vi "Database.WriteStationValues.vi"(8 "error in":errorcluster, 10 "FileName":string, 11 "Data in":T1 {"Variant"."TS"."TV"."minimum" format="%#.3f"; "Variant"."TS"."TV"."maximum" format="%#.3f"; "Variant"."TS"."TP"."value" format="%#.3f"}) -> (0 "error out":errorcluster, 3 "Data out":T1 {"Variant"."TS"."TV"."minimum" format="%#.3f"; "Variant"."TS"."TV"."maximum" format="%#.3f"; "Variant"."TS"."TP"."value" format="%#.3f"})   [LabVIEW 2016]
doc: "Write test results (measurement values) to proda database\n\nWabco 2017 All right reserved\nAuthor: maciej.szupienko@wabco-auto.com"
uses:
  tools/Translator/Translator.Message.ctl
  tools/EventLog/EventLog.EventSource.ctl
  Global/ApplicationGlobal.vi
  tools/EventLog/EventLog.New(single).vi
  Database.Main.Data.Sets.ctl
  Database.Main.Data.Status.ctl
  ProdaNG/Controls/ProdaNG.ProcessResult.ctl
  ProdaNG/Controls/ProdaNG.ProcessStepResult.ctl
  ProdaNG/Controls/ProdaNG.TestStepResult.ctl
  ProdaNG/Controls/ProdaNG.TestValueResult.ctl
  ProdaNG/Controls/ProdaNG.Identification.ctl
  Database.Main.Data.ctl
  Database.Main.Data.Results.ctl
  ProdaNG/Controls/ProdaNG.TestStepParam.ctl
  ProdaNG/Controls/ProdaNG.TestValue.ctl
  ProdaNG/Controls/ProdaNG.TestStep.ctl
  ProdaNG/Controls/ProdaNG.ProcessStepParam.ctl
  Database.Main.Data.Variant.ctl
panel:
  out "Prod saved":bool
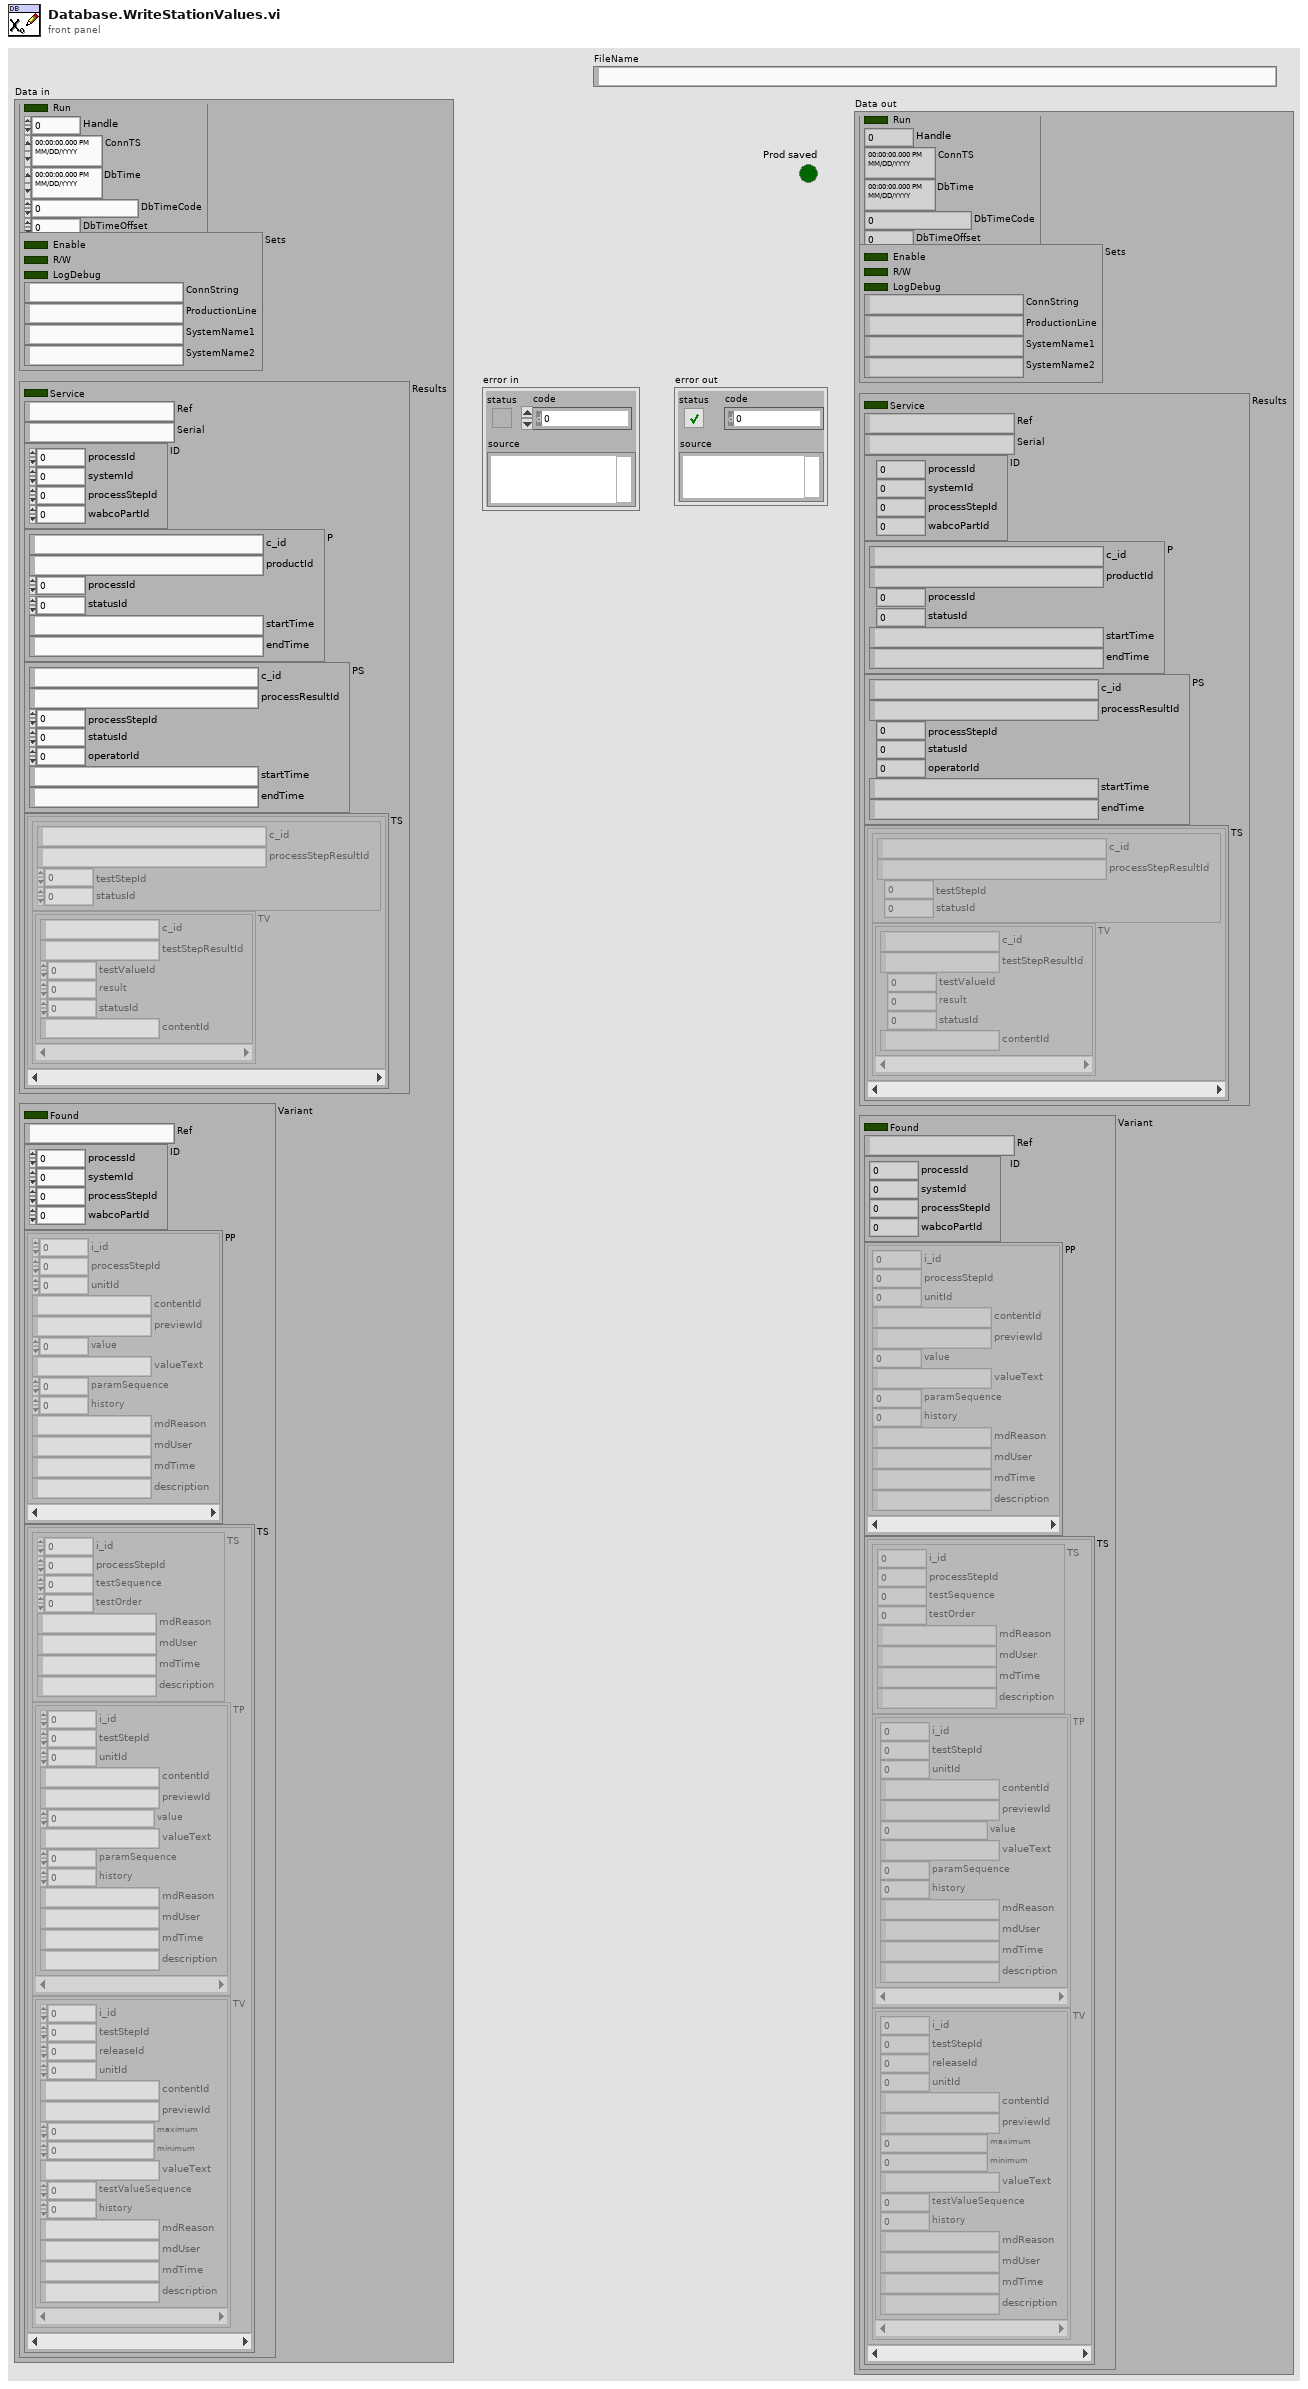
[diagram p1: front panel]
types:
  T1 = typedef "Database.Main.Data.ctl" = cluster{"Status":T2, "Sets":T3, "Results":T4, "Variant":T10}
  T2 = typedef "Database.Main.Data.Status.ctl" = cluster{"Run":bool, "Handle":i32, "ConnTS":timestamp, "DbTime":timestamp, "DbTimeCode":dbl, "DbTimeOffset":dbl}
  T3 = typedef "Database.Main.Data.Sets.ctl" = cluster{"Enable":bool, "R/W":bool, "LogDebug":bool, "ConnString":string, "ProductionLine":string, "SystemName1":string, "SystemName2":string}
  T4 = typedef "Database.Main.Data.Results.ctl" = cluster{"Service":bool, "Ref":string, "Serial":string, "ID":T5, "P":T6, "PS":T7, "TS":cluster{"TS":T8, "TV":T9[]}[]}
  T5 = typedef "ProdaNG.Identification.ctl" = cluster{"processId":i32, "systemId":i32, "processStepId":i32, "wabcoPartId":i32}
  T6 = typedef "ProdaNG.ProcessResult.ctl" = cluster{"c_id":string, "productId":string, "processId":i32, "statusId":i32, "startTime":string, "endTime":string}
  T7 = typedef "ProdaNG.ProcessStepResult.ctl" = cluster{"c_id":string, "processResultId":string, "processStepId":i32, "statusId":i32, "operatorId":i32, "startTime":string, "endTime":string}
  T8 = typedef "ProdaNG.TestStepResult.ctl" = cluster{"c_id":string, "processStepResultId":string, "testStepId":i32, "statusId":i32}
  T9 = typedef "ProdaNG.TestValueResult.ctl" = cluster{"c_id":string, "testStepResultId":string, "testValueId":i32, "result":dbl, "statusId":i32, "contentId":string}
  T10 = typedef "Database.Main.Data.Variant.ctl" = cluster{"Found":bool, "Ref":string, "ID":T5, "PP":T11[], "TS":cluster{"TS":T12, "TP":T13[], "TV":T14[]}[]}
  T11 = typedef "ProdaNG.ProcessStepParam.ctl" = cluster{"i_id":i32, "processStepId":i32, "unitId":i32, "contentId":string, "previewId":string, "value":dbl, "valueText":string, "paramSequence":i32, "history":i32, "mdReason":string, "mdUser":string, "mdTime":string, "description":string}
  T12 = typedef "ProdaNG.TestStep.ctl" = cluster{"i_id":i32, "processStepId":i32, "testSequence":i32, "testOrder":i32, "mdReason":string, "mdUser":string, "mdTime":string, "description":string}
  T13 = typedef "ProdaNG.TestStepParam.ctl" = cluster{"i_id":i32, "testStepId":i32, "unitId":i32, "contentId":string, "previewId":string, "value":dbl, "valueText":string, "paramSequence":i32, "history":i32, "mdReason":string, "mdUser":string, "mdTime":string, "description":string}
  T14 = typedef "ProdaNG.TestValue.ctl" = cluster{"i_id":i32, "testStepId":i32, "releaseId":i32, "unitId":i32, "contentId":string, "previewId":string, "maximum":dbl, "minimum":dbl, "valueText":string, "testValueSequence":i32, "history":i32, "mdReason":string, "mdUser":string, "mdTime":string, "description":string}
  T15 = typedef "EventLog.EventSource.ctl" = enum16{"All", "Gui", "Ref", "File", "Arch", "Seq", "CPX", "DB", "Laser", "Scan.P", "Scan.O"}
  T16 = typedef "Translator.Message.ctl" = enum16{"-", "Event confirmed", "Log out", "Log in", "Shutdown", "Cancel", "Start", "Begin time", "End time", "Duration", "Service Mode", "Ignore Results", "Serial Format", "On", "Off", "OK", "NOK", "NOK %s", "Home", "Work", "Close", "Open", "In progress...", "Missing", "Empty", "Hardware failure", "Initial", "Default", "Total", "Out of range", "Free disk space is below 1GB - contact technician", "Error %d >> %s", "Error %d >> %s >> %s", "Msg %d >> %s", "Laser msg %d %s", "Laser cmd error %s %d", "Laser cmd failed %s", "Laser cmd warning %s", "Laser disconnected", "Laser status %s", "Laser already started", "Laser job unkonwn %s", "Laser job missing %s", "Laser job select failure %s", "Unable to start laser printing (%s)", "Unable to stop laser printing (%s)", "Laser marking aborted", "Laser marking timeout", "Unable to reset Laser Interlock (%s)", "Unable to trigger Laser. Laser not ready (%s)", "Laser job '%s' coordinates not configured", "Starting %s", "Quitting %s", "Configured", "Initializing", "Quitting", "Loading", "Loaded %d results", "Loaded %d events", "Running", "Stopped", "Summary", "Laser", "Do you want to continue?", "Do you want to delete the configuration?", "The configuration is being used by an order. Unable to delete!", "Press confirm button", "Station is not based. Do you want to exit?", "Station requires changeover. Do you want to run the test?", "Test options are not set as default. Do you want to continue?", "Formatting of WabcoNo is disabled. Do you want to continue?", "Product not detected. Do you want to continue?", "Product scan failed. Do you want to continue?", "Calibration", "Log out?", "System", "All", "IDLE", "Translating...%s", "Not found", "Alarm %s", "Run", "Skip", "Abort", "Repeat", "Please wait...", "Database disconnected", "Database disconnected - changeover disabled!", "Login to database successful", "Login to database failed: %d; %s", "Unable to check the product status of reference %d - database disconnected", "Unable to set the product status of reference %d - database disconnected", "Variant file backup %s", "Read variant (%s)", "Result", "Station armed!", "Station requires changeover!", "Select reference number...", "EMERGENCY BUTTON - press Control button", "EMERGENCY DOOR - press Control button", "Resetting Emergency...", "Unable to reset safety circuit - Emergency Button pressed", "Unable to reset safety circuit - Emergency Side Door open", "Station not based", "Station based", "Station not empty", "Station basing...", "No order", "Press Start to begin new order", "Scanning new order", "Order NOK. Correct or scan again", "Order OK. Press Accept", "Order ready", "Revolver incorrect", "Fork incorrect", "Revolver missing", "Revolver empty", "Container missing", "Offline results", "Offline statistics", "Updating statistics %.1f %%", "DMC Configurator", "Door open", "Close the front door", "Press start button", "Done. Open the front door", "Running...", "Running...%.1f %%", "Pause %s", "Pause %s. NOK container missing", "Pause %s. OK container missing", "Pause %s. Revolver empty", "Pause %s. Revolver missing", "Pause %s. Revolver incorrect", "Pause %s. Fork missing", "Pause %s. Fork incorrect", "Pause %s. Too many failures", "Pause %s. Unloading failure", "Pause %s. One slot is not working", "Pause %s. Part order is done. Empty OK container", "Pause %s. Unable to move product to slot", "Pause %s. Unable to move back product pusher", "Pause %s. Unable to lift product", "Pause %s. Unable to move back product lifter", "Pause %s. Unable to move product arm to Work", "Pause %s. Unable to move product arm to NOK", "Pause %s. Unable to move product arm to OK", "Pause %s. Unable to unsuck the NOK product", "Pause %s. Unable to drop the NOK product", "Pause %s. Product OK missing", "Pause %s. Unable to unsuck the OK product", "Pause %s. Unable to drop the OK product", "Stopping...", "File '%s' is missing", "File '%s' is broken", "File '%s' is running", "Log file started (%s)", "Log file ended (%s)", "Log file stopped (%s)", "Log file ignored (%s)", "Log file exported (%s)", "Log file export failed (%s)", "Wrong serial number in log file", "Wrong reference number in log file", "Test steps are missing", "%s = %.3f", "Process param '%s' not found in DB", "Process param '%s' wrong order", "Process param '%s' value %.3f out of limits (%.3f; %.3f)", "Step%d param '%s' not found in DB", "Step%d param '%s' wrong order", "Step%d param '%s' value %.3f out of limits (%.3f; %.3f)", "Step%d EV '%s' not found in DB", "Step%d EV '%s' wrong order", "\"%s\" not found in DB", "\"%s\" wrong order", "\"%s\" value %.3f out of limits (%.3f; %.3f)", "\"%s\" not found in software", "Process init (%s)", "Process started", "Process restarted", "Process run", "Process done", "Process done - remove OK container", "Process aborted", "Process aborted at work", "Process aborted at home", "Process error", "Process error at home", "Process error at work", "Process close", "Process pause", "Process continue", "Process door open", "Process door close", "Process pause at slot %s due to %s", "Select plate from the order to process", "Do you want to start the process?", "Do you want to continue the process?", "There is unfinished order. Do you want to put the new order?", "Product %s %d OK", "Product %s %d NOK", "Unable to unload the slot %s. Product missing in the slot", "Unable to unload the slot %s. Product already in the arm", "Unable to accept the product as OK. Product missing in slot %s", "Unable to accept the product as OK. Product could not drop into the container at slot %s", "Unable to accept the product as NOK. Product could not drop into the container at slot %s", "Scan failed. Error %s", "Scan failed. Scanner disconnected", "Scan failed. Wrong Wabco number %d, limit (%d,%d)", "Scan failed. Wrong serial number %d, limit (%d,%d)", "Scan failed. Wrong date %d, limit (%d,%d)", "Scan failed. Wrong product wabco number %d (expected %d)", "Scan failed. Wrong product serial number %d (expected > 0)", "Scan OK %s", "Scan failed. Unable to determine table position (%s)", "Scan failed. Timeout", "Tune failed. Scanner disconnected", "Tune failed. Timeout", "%s = %d", "%s = %d->%d", "Unable to set %s = %.2f - Air Pressure Inside off", "Unable to set digital output '%s' = %d", "Unable to activate air pressure inside - timeout", "Unable to activate air pressure inside - aborted", "Unable to switch on Air Main Valve - Air Pressure Inlet off", "Unable to switch on Air Main Valve - Door open", "Unable to switch off Air Main Valve - timeout", "Unable to switch off Air Main Valve - aborted", "Unable to rotate Table - timeout", "Unable to rotate Table - aborted", "Unable to rotate Table - Product Move not in Home position", "Unable to rotate Table - Air Pressure Inside off", "Unable to rotate Table - Product Lift A not in Home position", "Unable to rotate Table - Product Lift B not in Home position", "Unable to rotate Table - unlock before movement timeout", "Unable to rotate Table - lock after movement timeout", "Unable to move Table Lock to %s position - timeout", "Unable to move Table Lock to %s position - aborted", "Unable to move Table Lock to %s position - Air Pressure Inside off", "Unable to move Table Lock to %s position - Table not in position", "Unable to move Product Lift A to %s position - timeout", "Unable to move Product Lift B to %s position - timeout", "Unable to move Product Lift A to %s position - aborted", "Unable to move Product Lift B to %s position - aborted", "Unable to move Product Lift A to %s position - Air Pressure Inside off", "Unable to move Product Lift B to %s position - Air Pressure Inside off", "Unable to move Product Lift A to %s position - Table not locked", "Unable to move Product Lift B to %s position - Table not locked", "Unable to move Product Lift A to %s position - Product Arm not in Work position", "Unable to move Product Lift B to %s position - Product Arm not in Work position", "Unable to set Product Suction Gripper %s to %s - timeout", "Unable to set Product Suction Gripper %s to %s - aborted", "Unable to set Product Suction Gripper %s to %s - Air Pressure Inside off", "Unable to set Product Suction Gripper %s to %s - Table slot unkown", "Unable to move Product Arm to %s position - timeout", "Unable to move Product Arm to %s position - aborted", "Unable to move Product Arm to %s position - Air Pressure Inside off", "Unable to move Product Arm to %s position - Product Lift A not in Home position", "Unable to move Product Arm to %s position - Product Lift B not in Home position", "Unable to move Product to %s position - timeout", "Unable to move Product to %s position - aborted", "Unable to move Product to %s position - Air Pressure Inside off", "Unable to move Product to %s position - Table not in position"}
  T17 = typedef "Logger.File.ctl" = cluster{"Props":T18, "Data":T21[]}
  T18 = typedef "Logger.File.Properties.ctl" = cluster{"FilePath":path, "ImgFolder":string, "Ref":string, "Serial":string, "SerialFormat":T19, "Duration":dbl, "Time From":timestamp, "Time To":timestamp, "Service":bool, "IgnoreImgs":bool, "CheckDMC":bool, "Counters":T20, "Err":errorcluster}
  T19 = typedef "Sequence.Code.SerialFormat.ctl" = enum8{"", "6 dig", "7 dig"}
  T20 = typedef "Sequence.Counters.ctl" = cluster{"Expected":u16, "Done":u16, "OK":u16, "NOK":u16, "NOKlimit":u16, "Part":u16, "PartOK":u16}
  T21 = typedef "Logger.File.Serials.ctl" = cluster{"TS from":timestamp, "TS to":timestamp, "SlotID":u8, "StatusA":T22, "SerialA":string, "CodeA":string, "ImgA":string, "CornersA":cluster{"X":i32, "Y":i32}[], "verificationA":u8, "StatusB":T22, "SerialB":string, "CodeB":string, "ImgB":string, "CornersB":cluster{"X":i32, "Y":i32}[], "verificationB":u8}
  T22 = typedef "Sequence.Step.Status.ctl" = enum16{"-", "Pending", "Running", "Skipped", "Passed", "Failed", "Done", "Error", "Aborted", "Stopped"}
  T23 = cluster{"date/time string":string, "date/time string":string, "StatusA":T22, "SerialA":string}
  T24 = cluster{"date/time string":string, "date/time string":string, "StatusB":T22, "SerialB":string}
  T25 = cluster{"date/time string":string, "date/time string":string, "StatusB":T22, "SerialB":string}[]
  T26 = typedef "ProdaNG.Product.ctl" = cluster{"c_id":string, "wabcoPartId":i32, "serialNumber":string, "comment":string, "individual":i32, "crProcessStepId":i32, "mdProcessStepId":i32, "crTime":string, "mdTime":string}
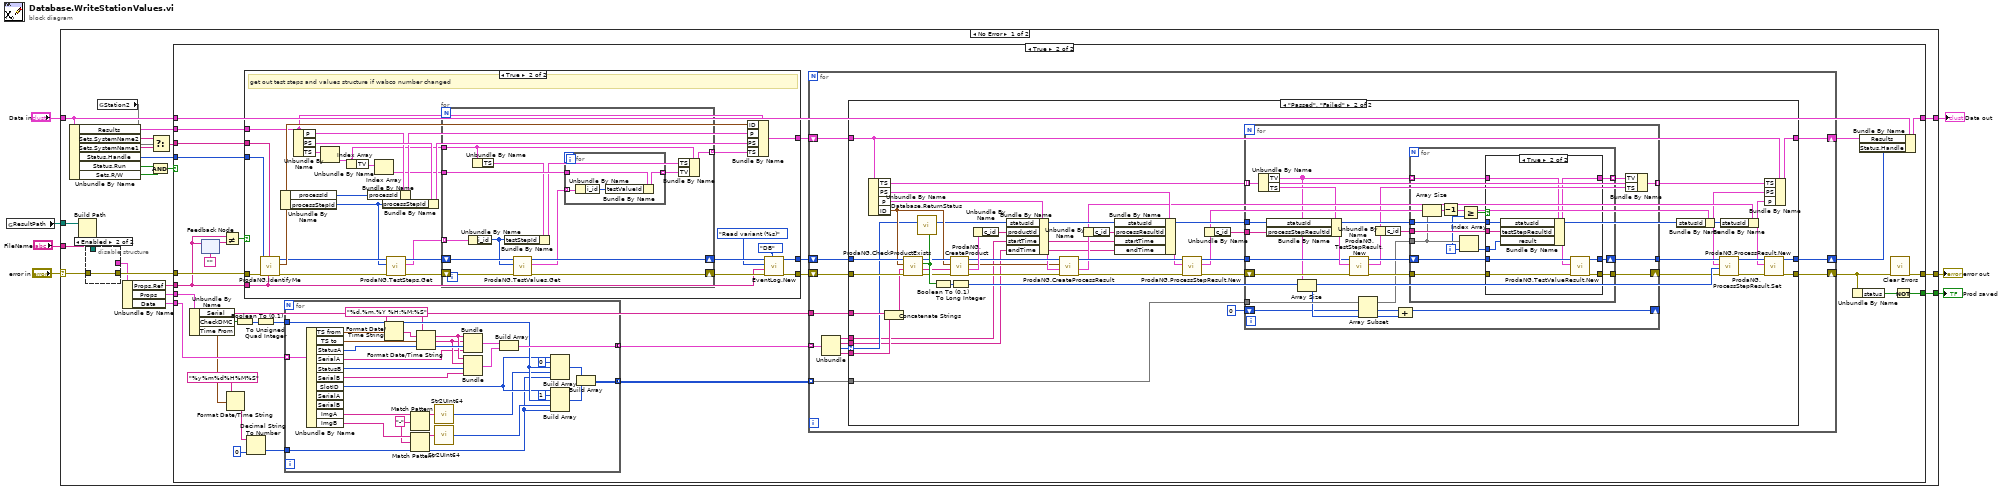
[diagram p0: block diagram]
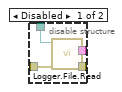
[diagram p2: hidden frame]
diagram:
  n1 = global read "ApplicationGlobal.vi" "ResultPath"() -> (w2:path)
  n2 = case shown="No Error" "error in" {
    selector: "error in" -> [w13 w254]
    tunnel: [w25 w254] -> w7
    tunnel: "Data in" -> [w28 w253]
    tunnel: [w27 w253] -> w4
    tunnel: [w23 _] -> w3
    tunnel: w2 -> [w16 _]
    tunnel: "FileName" -> [w15 _]
    frame No Error {
      n3 = Unbundle By Name(w28) -> ("Results"=w26:T4, "Sets.SystemName2"=w20:string, "Sets.SystemName1"=w19:string, "Status.Handle"=w29:i32, "Status.Run"=w24:bool, "Sets.R/W"=w21:bool)
      n4 = Build Path(base path=w16, name or relative path=w15) -> (appended path=w14:path)
      n5 = disable-structure shown="Enabled" {
        disable-tunnel: w14 -> [w33 _]
        disable-tunnel: w13 -> [w32 w34]
        disable-tunnel: [w31 w34] -> w12
        disable-tunnel: [w30 _] -> w11
        frame Disabled {
          n6 = call "Logger.File.Read.vi"("error in (no error)"=w32, "file path"=w33) -> ("error out"=w31:errorcluster, "File content"=w30:T17)  [unwired: 6 in, 2 out]
        }
        frame Enabled {
        }
      }
      n7 = global read "ApplicationGlobal.vi" "Station2"() -> (w18)
      n8 = Unbundle By Name(w11) -> ("Props.Ref"=w10:string, "Props"=w8:T18, "Data"=w9:T21[])
      n9 = Select(t=w20, s=w18, f=w19) -> (s? t:f=w17:string)
      n10 = Compound Arithmetic op=AND(w24, w21) -> (w22:bool)
      n11 = case shown="True" w22 {
        tunnel: w12 -> [w36 w68]
        tunnel: w17 -> [_ w67]
        tunnel: w29 -> [_ w66]
        tunnel: w10 -> [_ w58]
        tunnel: w28 -> [w35 w65]
        tunnel: [w35 w64] -> w27
        tunnel: w26 -> [_ w63]
        tunnel: [w36 w50] -> w25
        tunnel: [_ w51] -> w23
        tunnel: w9 -> [_ w44]
        tunnel: w8 -> [_ w49]
        frame False {
        }
        frame True {
          n12 = Unbundle By Name(w49) -> ("Serial"=w48:string, "CheckDMC"=w47:bool, "Time From"=w40:timestamp)
          n13 = feedback #1("") -> (w60:string)
          n14 = feedback-in #1(w58) -> ()
          n15 = Not Equal?(x=w58, y=w60) -> (x != y?=w59:bool)
          n16 = Format Date/Time String(time format string (%c)="%y%m%d%H%M%S", seconds (now)=w40) -> (date/time string=w39:string)  [unwired: 1 in]
          n17 = Boolean To (0,1)(Boolean=w47) -> (0, 1=w46:i16)
          n18 = case shown="True" w59 {
            tunnel: w58 -> [_ w218]
            tunnel: w68 -> [w207 w225]
            tunnel: [w207 w221] -> w62
            tunnel: w67 -> [_ w223]
            tunnel: w66 -> [w206 w224]
            tunnel: [w206 w217] -> w61
            tunnel: w63 -> [w205 w215]
            tunnel: [w205 w222] -> w54
            frame False {
            }
            frame True {
              # "get out test steps and values structure if wabco number changed"
              n19 = call "ProdaNG.IdentifyMe.vi"("wabcoNumber"=w218, "systemName"=w223, "error in"=w225, "dbHandleIn"=w224) -> ("error out"=w226:errorcluster, "Identification"=w234:T5, "dbHandle"=w227:i32)  [unwired: 5 in]
              n20 = Unbundle By Name(w234) -> ("processId"=w229:i32, "processStepId"=w214:i32)
              n21 = Unbundle By Name(w215) -> ("P"=w232:T6, "PS"=w233:T7, "TS"=w212:cluster{"TS":T8, "TV":T9[]}[])
              n22 = Index Array(array=w212) -> (element=w209:cluster{"TS":T8, "TV":T9[]})  [unwired: 1 in]
              n23 = Unbundle By Name(w209) -> ("TV"=w211:T9[])
              n24 = Bundle By Name(cluster=w232, "processId"=w229) -> (w230:T6)
              n25 = Index Array(array=w211) -> (element=w210:T9)  [unwired: 1 in]
              n26 = Bundle By Name(cluster=w233, "processStepId"=w214) -> (w231:T7)
              n27 = call "ProdaNG.TestSteps.Get.vi"("error in (no error)"=w226, "processStepId"=w214, "dbHandleIn"=w227) -> ("error out"=w228:errorcluster, "TestSteps"=w213:T12[], "dbHandle"=w235:i32)  [unwired: 6 in]
              n28 = for {
                tunnel: w213 -> [w243] mode=indexing
                tunnel: w210 -> [w241]
                shift-right: [w245] -> w217
                shift-left: w235 -> [w248]
                shift-right: [w246] -> w220
                shift-left: w228 -> [w247]
                tunnel: w209 -> [w239]
                tunnel: [w236] -> w208 mode=indexing
                n29 = Unbundle By Name(w243) -> ("i_id"=w242:i32)
                n30 = Unbundle By Name(w239) -> ("TS"=w238:T8)
                n31 = Bundle By Name(cluster=w238, "testStepId"=w242) -> (w237:T8)
                n32 = call "ProdaNG.TestValues.Get.vi"("error in (no error)"=w247, "testStepId"=w242, "dbHandleIn"=w248) -> ("error out"=w246:errorcluster, "TestStepValues"=w244:T14[], "dbHandle"=w245:i32)  [unwired: 6 in]
                n33 = for {
                  tunnel: w244 -> [w252] mode=indexing
                  tunnel: w241 -> [w250]
                  tunnel: [w249] -> w240 mode=indexing
                  n34 = Unbundle By Name(w252) -> ("i_id"=w251:i32)
                  n35 = Bundle By Name(cluster=w250, "testValueId"=w251) -> (w249:T9)
                }
                n36 = Bundle By Name(cluster=w239, "TS"=w237, "TV"=w240) -> (w236:cluster{"TS":T8, "TV":T9[]})
              }
              n37 = Bundle By Name(cluster=w215, "ID"=w234, "P"=w230, "PS"=w231, "TS"=w208) -> (w222:T4)
              n38 = call-poly "EventLog.New.vi"("Source (All)"=EventLog.EventSource."DB", "error in (no error)"=w220, "Arg"=w218, "Message (-)"=Translator.Message."Read variant (%s)") -> ("error out"=w221:errorcluster)  [unwired: 6 in, 1 out]
            }
          }
          n39 = Decimal String To Number(string=w39, default (0L)=u64 0 ("default (0 I32)")) -> (number=w37:u64)  [unwired: 1 in, 1 out]
          n40 = To Unsigned Quad Integer(1:w46) -> (0:w45:u64)
          n41 = for {
            tunnel: w44 -> [w96] mode=indexing
            tunnel: [w92] -> w43 mode=concatenating
            tunnel: w45 -> [w88]
            tunnel: [w86] -> w42 mode=concatenating
            tunnel: w37 -> [w69]
            w72 = "%d.%m.%Y %H:%M:%S" ("time format string (%c)")
            w83 = "-" ("regular expression")
            n42 = Unbundle By Name(w96) -> ("TS from"=w80:timestamp, "TS to"=w79:timestamp, "StatusA"=w95:T22, "SerialA"=w71:string, "StatusB"=w94:T22, "SerialB"=w70:string, "SlotID"=w76:u8, "ImgA"=w75:string, "ImgB"=w84:string)  [unwired: 2 out]
            n43 = Format Date/Time String(time format string (%c)=w72, seconds (now)=w80) -> (date/time string=w78:string)  [unwired: 1 in]
            n44 = Match Pattern(string=w75, regular expression=w83) -> (before substring=w85:string)  [unwired: 1 in, 3 out]
            n45 = Match Pattern(string=w84, regular expression=w83) -> (before substring=w82:string)  [unwired: 1 in, 3 out]
            n46 = Format Date/Time String(time format string (%c)=w72, seconds (now)=w79) -> (date/time string=w77:string)  [unwired: 1 in]
            n47 = call "Str2UInt64.vi"("string"=w85) -> ("Numeric"=w73:u64)
            n48 = call "Str2UInt64.vi"("string"=w82) -> ("Numeric"=w74:u64)
            n49 = Bundle("date/time string"=w78, "date/time string"=w77, "StatusA"=w95, "SerialA"=w71) -> (w93:T23)  [unwired: 1 in]
            n50 = Bundle("date/time string"=w78, "date/time string"=w77, "StatusB"=w94, "SerialB"=w70) -> (w91:T24)  [unwired: 1 in]
            n51 = Build Array(w93, w91) -> (w92:T25)
            n52 = Build Array(w76, u64 0, w88, w73, w69) -> (w81:u64[])
            n53 = Build Array(w76, u64 1, w88, w74, w69) -> (w87:u64[])
            n54 = Build Array(w81, w87) -> (w86:u64[][])
          }
          n55 = for {
            shift-right: [w104] -> w53
            shift-left: w62 -> [w109]
            shift-right: [w106] -> w55
            shift-left: w61 -> [w108]
            shift-right: [w107] -> w56
            shift-left: w54 -> [w105]
            tunnel: w48 -> [w102]
            tunnel: w43 -> [w103] mode=indexing
            tunnel: w42 -> [w101] mode=indexing
            n56 = Unbundle(w103) -> ("date/time string"=w98:string, "date/time string"=w99:string, "StatusB"=w97:T22, "SerialB"=w100:string)
            n57 = case shown="\"Passed\", \"Failed\"" w97 {
              selector: w97 -> [_ w117]
              tunnel: w109 -> [w112 w137]
              tunnel: w108 -> [w111 w136]
              tunnel: [w110 w127] -> w107
              tunnel: [w111 w123] -> w106
              tunnel: w105 -> [w110 w122]
              tunnel: [w112 w121] -> w104
              tunnel: w102 -> [_ w119]
              tunnel: w100 -> [_ w118]
              tunnel: w101 -> [_ w116]
              tunnel: w99 -> [_ w114]
              tunnel: w98 -> [_ w115]
              frame Default {
              }
              frame "Passed", "Failed" {
                n58 = Unbundle By Name(w122) -> ("TS"=w134:cluster{"TS":T8, "TV":T9[]}[], "PS"=w133:T7, "P"=w132:T6, "ID"=w131:T5)
                n59 = Concatenate Strings(w119, w118) -> (w113:string)
                n60 = call "ProdaNG.CheckProductExists.vi"("error in (no error)"=w137, "serialNumber"=w113, "ID"=w131, "dbHandle"=w136) -> ("error out"=w139:errorcluster, "Results exist?"=w157:bool, "dbHandle out"=w135:i32)  [unwired: 2 in, 3 out]
                n61 = call "Database.ReturnStatus.vi"("repeat"=w157, "Status"=w117) -> ("Step.statusId"=w130:i32)  [unwired: 8 in, 1 out]
                n62 = Boolean To (0,1)(Boolean=w157) -> (0, 1=w138:i16)
                n63 = call "ProdaNG.CreateProduct.vi"("error in (no error)"=w139, "serialNumber"=w113, "ID"=w131, "dbHandle"=w135) -> ("error out"=w151:errorcluster, "Product out"=w156:T26, "dbHandle out"=w152:i32)  [unwired: 4 in, 1 out]
                n64 = To Long Integer(number=w138) -> (32bit integer=w155:i32)
                n65 = Unbundle By Name(w156) -> ("c_id"=w142:string)
                n66 = Bundle By Name(cluster=w132, "statusId"=w130, "productId"=w142, "startTime"=w115, "endTime"=w114) -> (w150:T6)
                n67 = call "ProdaNG.CreateProcessResult.vi"("error in (no error)"=w151, "ProcessResult"=w150, "ID"=w131, "dbHandle"=w152) -> ("error out"=w153:errorcluster, "ProcessResult 2"=w128:T6, "dbHandle out"=w154:i32)  [unwired: 5 in]
                n68 = Unbundle By Name(w128) -> ("c_id"=w143:string)
                n69 = Bundle By Name(cluster=w133, "statusId"=w130, "processResultId"=w143, "startTime"=w115, "endTime"=w114) -> (w149:T7)
                n70 = call "ProdaNG.ProcessStepResult.New.vi"("error in (no error)"=w153, "ProcessStepResult"=w149, "dbHandle"=w154) -> ("error out"=w141:errorcluster, "ProcessStepResult out"=w125:T7, "dbHandle"=w140:i32)  [unwired: 6 in]
                n71 = Unbundle By Name(w125) -> ("c_id"=w144:string)
                n72 = for {
                  tunnel: [w177] -> w146
                  tunnel: w144 -> [w175]
                  tunnel: w140 -> [w173]
                  tunnel: w116 -> [w163]
                  tunnel: w134 -> [w168] mode=indexing
                  tunnel: w130 -> [w169]
                  tunnel: [w164] -> w129 mode=indexing
                  shift-right: [w176] -> w145
                  shift-left: w141 -> [w174]
                  shift-right: [w158] -> _
                  shift-left: 0 -> [w160]
                  n73 = Unbundle By Name(w168) -> ("TV"=w162:T9[], "TS"=w166:T8)
                  n74 = Bundle By Name(cluster=w166, "statusId"=w169, "processStepResultId"=w175) -> (w178:T8)
                  n75 = Array Size(array=w162) -> (size(s)=w161:i32)
                  n76 = call "ProdaNG.TestStepResult.New.vi"("error in (no error)"=w174, "TestStepResult"=w178, "dbHandle"=w173) -> ("error out"=w170:errorcluster, "TestStepResult out"=w165:T8, "dbHandle"=w171:i32)  [unwired: 6 in]
                  n77 = Array Subset(array=w163, index=w160, length=w161) -> (w159:u64[])
                  n78 = Unbundle By Name(w165) -> ("c_id"=w172:string)
                  n79 = Compound Arithmetic op=ADD(w160, w161) -> (w158:i32)
                  n80 = for "results" {
                    tunnel: w170 -> [w192]
                    tunnel: [w189] -> w176
                    tunnel: w172 -> [w190]
                    shift-right: [w188] -> w177
                    shift-left: w171 -> [w191]
                    tunnel: w159 -> [w183]
                    tunnel: w169 -> [w187]
                    tunnel: w162 -> [w186] mode=indexing
                    tunnel: [w185] -> w167 mode=indexing
                    i -> [w181]
                    n81 = Array Size(array=w183) -> (size(s)=w180:i32)
                    n82 = Decrement(x=w180) -> (x-1=w179:i32)
                    n83 = Index Array(array=w183, index=w181) -> (element=w184:u64)
                    n84 = Greater Or Equal?(x=w179, y=w181) -> (x >= y?=w182:bool)
                    n85 = case shown="True" w182 {
                      tunnel: w192 -> [w194 w204]
                      tunnel: w191 -> [w193 w203]
                      tunnel: w190 -> [_ w202]
                      tunnel: [w194 w201] -> w189
                      tunnel: [w193 w200] -> w188
                      tunnel: w187 -> [_ w199]
                      tunnel: w186 -> [w195 w198]
                      tunnel: [w195 w197] -> w185
                      tunnel: w184 -> [_ w196]
                      frame False {
                      }
                      frame True {
                        n86 = Bundle By Name(cluster=w198, "statusId"=w199, "testStepResultId"=w202, "result"=w196) -> (w197:T9)
                        n87 = call "ProdaNG.TestValueResult.New.vi"("error in (no error)"=w204, "TestValueResult"=w197, "dbHandle"=w203) -> ("error out"=w201:errorcluster, "dbHandle"=w200:i32)  [unwired: 7 in]
                      }
                    }
                  }
                  n88 = Bundle By Name(cluster=w168, "TV"=w167, "TS"=w165) -> (w164:cluster{"TS":T8, "TV":T9[]})
                }
                n89 = Bundle By Name(cluster=w125, "statusId"=w130) -> (w124:T7)
                n90 = call "ProdaNG.ProcessStepResult.Set.vi"("error in (no error)"=w145, "isRepeat (0)"=w155, "ProcessStepResult"=w124, "dbHandle"=w146) -> ("error out"=w148:errorcluster, "dbHandle"=w147:i32)  [unwired: 6 in]
                n91 = Bundle By Name(cluster=w128, "statusId"=w130) -> (w126:T6)
                n92 = Bundle By Name(cluster=w122, "TS"=w129, "PS"=w124, "P"=w126) -> (w127:T4)
                n93 = call "ProdaNG.ProcessResult.New.vi"("error in (no error)"=w148, "ProcessResult"=w126, "dbHandle"=w147) -> ("error out"=w121:errorcluster, "dbHandle"=w123:i32)  [unwired: 6 in, 1 out]
              }
            }
          }
          n94 = Unbundle By Name(w53) -> ("status"=w52:bool)
          n95 = Bundle By Name(cluster=w65, "Results"=w56, "Status.Handle"=w55) -> (w64:T1)
          n96 = call <vilib>:"Clear Errors.vi"("error in (no error)"=w53) -> ("error out"=w50:errorcluster)  [unwired: 5 in, 1 out]
          n97 = Not(x=w52) -> (.not. x?=w51:bool)
        }
      }
    }
    frame Error {
    }
  }
  "error out" <- w7
  "Prod saved" <- w3
  "Data out" <- w4
